vi "Strip.vi"(9 "Regex":string, 11 "Input String":string) -> (2 "Result String":string)   [LabVIEW 2011]
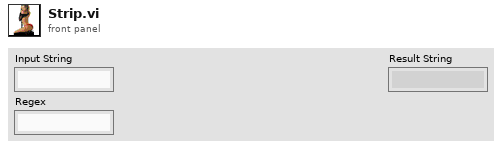
[diagram p1: front panel]
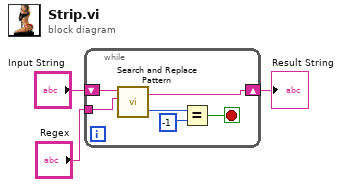
[diagram p0: block diagram]
diagram:
  n1 = while {
    shift-right: [w6] -> w2
    shift-left: "Input String" -> [w5]
    tunnel: "Regex" -> [w4]
    stop <- w7 stop-if-true
    n2 = call <vilib>:"Search and Replace Pattern.vi"("string"=w5, "regular expression (\"\")"=w4) -> ("result string"=w6:string, "offset past match"=w9:i32)  [unwired: 3 in]
    n3 = Equal?(x=w9, y=-1) -> (x = y?=w7:bool)
  }
  "Result String" <- w2
